vi "GetCString_byPtr.vi"(5 "error in (no error)":errorcluster, 7 "MaxSize":i32=1000, 8 "C String Pointer":i32) -> (0 "error out":errorcluster, 2 "String":string, 3 "Duplicate Pointer":i32)   [LabVIEW 2011]
doc: "Use this VI to return any C String (NULL terminated) from memory using a pointer. This VI may cause problems if used to read memory which is not Null terminated. Use the <B>Max Size</B> input to help protect against this. If the VI reads a string larger than <B>Max Size</B> it will return a string overrun error.\n\n*Warning - The pointer VIs access memory directly. The VIs will check for NULL pointers, but may still cause access violations and crashes if used to access protected or otherwise inaccessible memory locations."
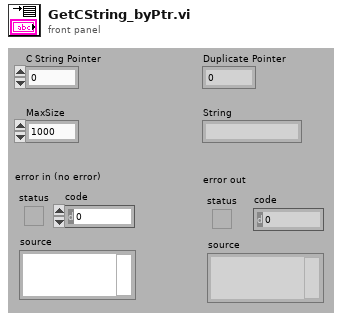
[diagram p1: front panel]
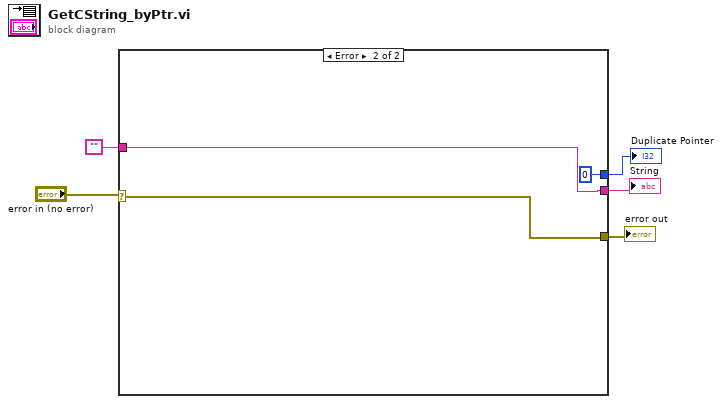
[diagram p0: block diagram]
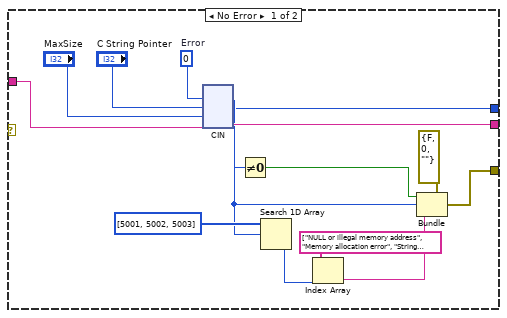
[diagram p2: hidden frame]
diagram:
  n1 = case shown="Error" "error in (no error)" {
    selector: "error in (no error)" -> [_ w22]
    tunnel: [w10 w21] -> w4
    tunnel: [w13 w22] -> w3
    tunnel: "" -> [w9 w21]
    tunnel: [w6 0 ("C String Pointer")] -> w1
    frame No Error {
      w8 = 0  # Error
      n2 = cin(w8, "C String Pointer", "MaxSize", w9) -> (w7:i32, w6:i32, w10:string)  [unwired: 1 in]
      n3 = Not Equal To 0?(x=w7) -> (x != 0?=w18:bool)
      n4 = Search 1D Array(1D array=i32[] [5001, 5002, 5003], element=w7) -> (index of element=w16:i32)  [unwired: 1 out]
      n5 = Index Array(array=string[] ["NULL or illegal memory address", "Memory allocation error", "String overrun"], index=w16) -> (element=w14:string)
      n6 = Bundle(cluster=errorcluster {"status"=FALSE, "code"=0, "source"=""} ("error IO"), "status"=w18, "code"=w7, "source"=w14) -> (w13:errorcluster)
    }
    frame Error {
    }
  }
  "error out" <- w3
  "String" <- w4
  "Duplicate Pointer" <- w1
